vi "ZeroE4418B.vi"(2 "error in (no error)":errorcluster) -> (0 "error out":errorcluster)   [LabVIEW 2009]
doc: "Zero the E4418B power meter with zero input power"
panel:
  in  "SCPI zero commands":string="*cls\ncal:zero:auto once\n\n\n\n"
  # "Zero the E4418B power meter with zero input power."
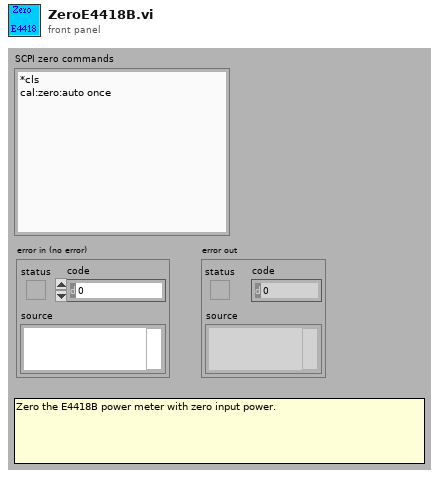
[diagram p1: front panel]
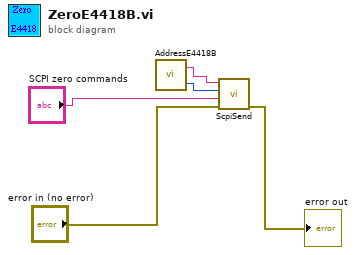
[diagram p0: block diagram]
diagram:
  n1 = call "AddressE4418B.vi"() -> ("Port"=w5:i32, "IP address"=w4:string)  [unwired: 2 in]
  n2 = call "ScpiSend.vi"("error in (no error)"="error in (no error)", "Command"="SCPI zero commands", "TCP port"=w5, "IP Address"=w4) -> ("error out"=→"error out":errorcluster)  [unwired: 7 in]
